vi "Dashboard Main.vi"() -> ()   [LabVIEW 2018]
uses:
  <vilib>/Utility/miscctls.llb/LVRowAndColumnTypeDef.ctl
  <vilib>/event_ctls.llb/eventvkey.ctl
  <vilib>/Rock Robotics/WPI/Dashboard/WPI_DashboardLogging Global.vi
  <vilib>/Rock Robotics/Network Tables/NT Read Numeric Array.vi
  <vilib>/Utility/inputDevices.llb/keyboardAcquire.vi
panel:
  in  "Camera Settings Right":T1={"Frame Rate"=30, "Compression"=30, "Size"=1, "DB Camera Config"=FALSE} {"Frame Rate" scale=1.0..30.0; "Compression" scale=100.0..-1.0; "Size" items=["640x480", "320x240", "160x120"]}
  in  "Camera Name Right":string(combo)="No Camera Selection"
  out "Camera Perf":string
  in  "Camera Settings":T1={"Frame Rate"=30, "Compression"=30, "Size"=1, "DB Camera Config"=FALSE} {"Frame Rate" scale=1.0..30.0; "Compression" scale=100.0..-1.0; "Size" items=["640x480", "320x240", "160x120"]}
  in  "TCP":refnum<k5>
  in  "Rec Mode":enum32{"Stop", "Record", "Playback"}(radio)
  out "Robot IP":string
  out "Image Message":string="Timeout in Camera Communications"
  in  "Dashboard Tab":T2(tab)
  in  "Select Auto":string(combo)="Select Autonomous ..."
  out "NT Connection":bool
  out "MotorChart R":cluster{"Numeric":dbl, "Numeric":dbl}(graph)
  out "MotorChart L":cluster{"Numeric":dbl, "Numeric":dbl}(graph)
  out "MotorSliders R":cluster{"MotorSlide1":dbl, "MotorSlide2":dbl} {"MotorSlide2" scale=-1.0..1.0 scale format="%#_2e"; "MotorSlide1" scale=-1.0..1.0 scale format="%#_2e"}
  out "MotorSliders L":cluster{"MotorSlide1":dbl, "MotorSlide2":dbl} {"MotorSlide2" scale=-1.0..1.0 scale format="%#_2e"; "MotorSlide1" scale=-1.0..1.0 scale format="%#_2e"}
  out "Gyro":dbl(knob) scale=0.0..360.0
  out "JS1 Z":dbl(slide) scale=-1.0..1.0 scale format="%#_2e"
  out "JS1 Graph":cluster{"X":dbl, "Y":dbl}[](graph)
  out "JS1 Buttons":T3
  out "JS2 Z":dbl(slide) scale=-1.0..1.0 scale format="%#_2e"
  out "JS2 Graph":cluster{"X":dbl, "Y":dbl}[](graph)
  out "JS2 Buttons":T3
  out "Mode":T4(ring)=enum."Auto Disabled"
  out "Right Camera Perf":cluster{"Bandwidth (Mbps)":dbl, "FPS":dbl}
  out "Camera Image Right":T5(plugin-control)
  in  "DB/String 9":string
  in  "DB/String 8":string
  in  "DB/String 7":string
  in  "DB/String 6":string
  in  "DB/String 5":string
  in  "DB/String 4":string
  in  "DB/String 3":string
  in  "DB/String 2":string
  in  "DB/String 1":string
  in  "DB/String 0":string
  in  "DB/Slider 0":dbl(slide) scale=0.0..5.0
  in  "DB/Slider 1":dbl(slide) scale=0.0..5.0
  in  "DB/Slider 2":dbl(slide) scale=0.0..5.0
  in  "DB/Slider 3":dbl(slide) scale=0.0..5.0
  out "DB/LED 3":bool
  out "DB/LED 2":bool
  out "DB/LED 1":bool
  out "DB/LED 0":bool
  in  "DB/Button 3":bool
  in  "DB/Button 2":bool
  in  "DB/Button 1":bool
  in  "DB/Button 0":bool caption="New Name"
  in  "Remove Point":bool
  in  "Add Point":bool
  out "XY Graph":cluster{"X":dbl, "Y":dbl}[](graph)
  in  "Interpolation Method":i32(ring)=1 items=["nearest", "linear", "spline", "cubic Hermite", "Lagrange"]
  in  "Test Slider":dbl(slide) scale=0.0..100.0 scale format="%#_3g"
  in  "On/Off":bool caption="Solenoid"
  in  "Test Name":u16(ring) items=["Select the test to run..."]
  in  "Test Tree":string(tree)
  in  "Motor":cluster{"Value":dbl, "Enable":bool} {"Value" scale=-1.0..1.0 scale format="%#_3g"}
  out "Progress":T6 {"Test Progress" scale=0.0..100.0}
  in  "Rev/Fwd":cluster{"Forward":bool, "Reverse":bool}
  in  "Test Ring":u16(ring) items=["Monochrome", "Color"]
  out "Cmd Status":string
  in  "Execute Command":bool
  in  "Command Params":string[][](table)
  in  "Command Selection":i32(listbox)
  in  "CheckList":i32(listbox)
  out "Tree":string(tree)
  out "Camera Image":T5(plugin-control)
  out "Background":bool
  in  "Camera Name":string(combo)="No Camera Selection"
  # "HW"
  # "HW"
  # "Joysticks"
  # "Raw Input"
  # "Proccessed"
  # "Drive Motors"
  # "Front"
  # "Right"
  # "Left"
  # "Back"
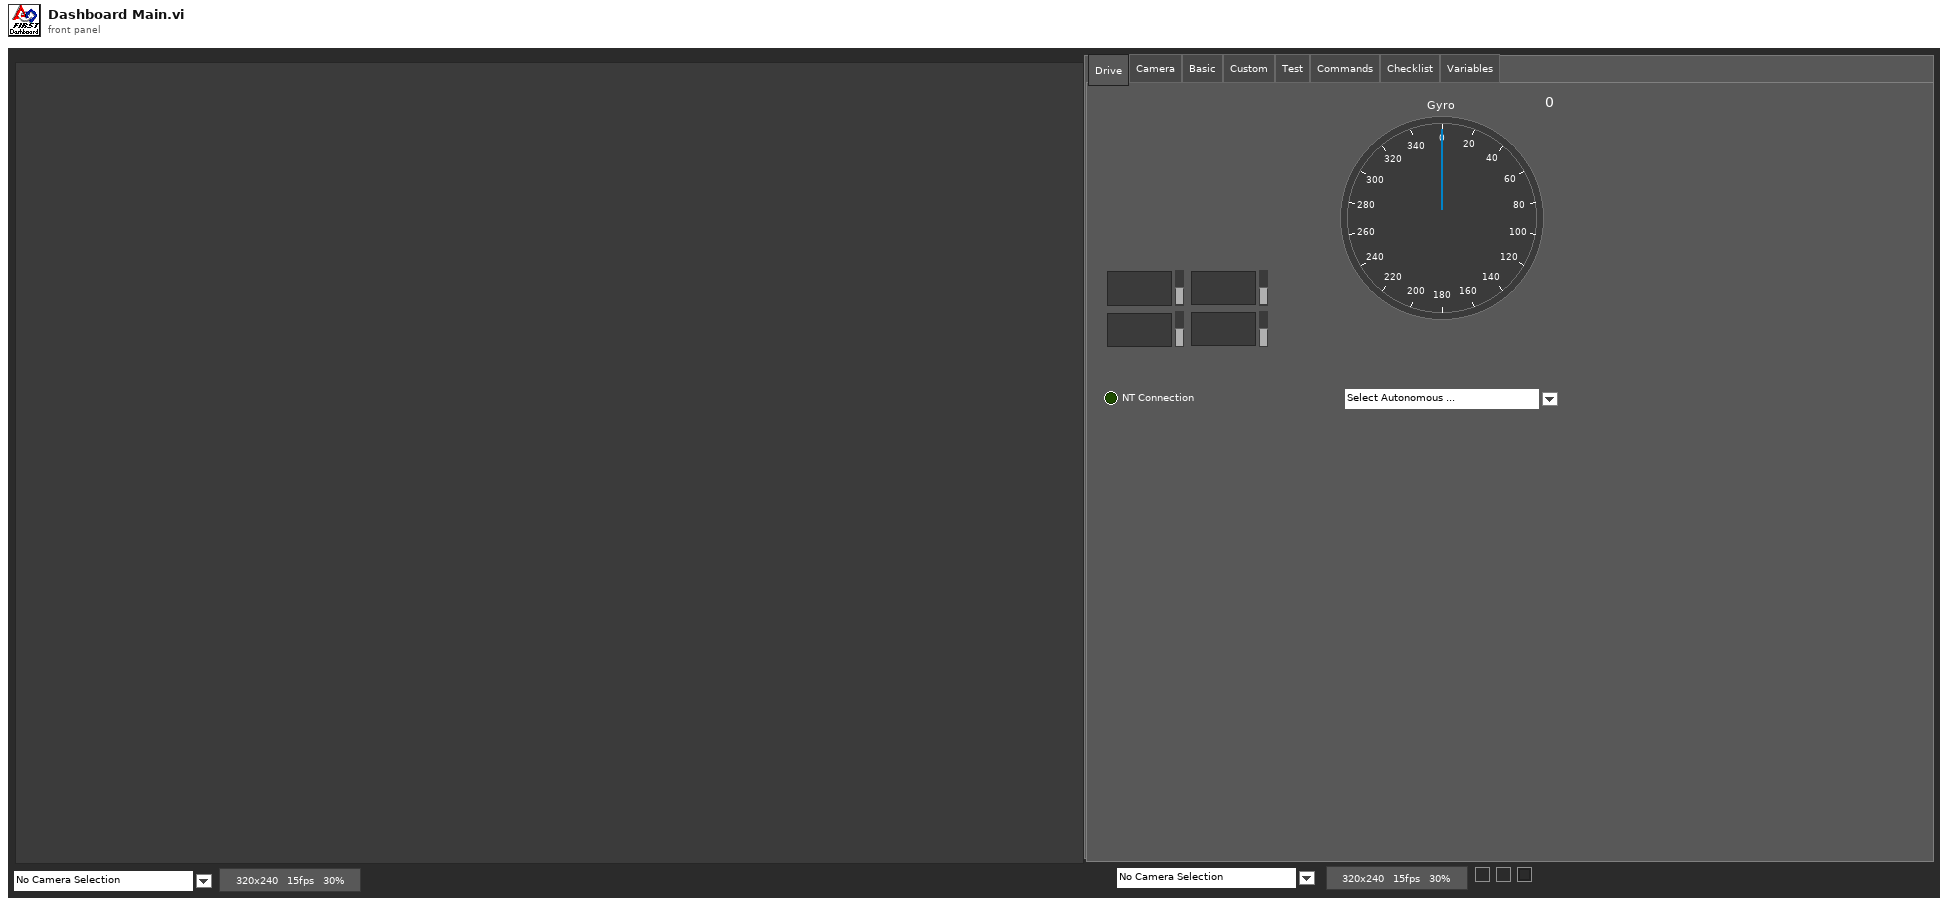
[diagram p1: front panel]
types:
  T1 = cluster{"Frame Rate":i32, "Compression":i32, "Size":u16, "DB Camera Config":bool}
  T2 = enum32{"Drive", "Camera", "Basic", "Custom", "Test", "Commands", "Checklist", "Variables"}
  T3 = cluster{bool, bool, bool, bool, bool, bool, bool, bool, bool, bool, bool, bool}
  T4 = enum8{"Tele-Op Disabled", "Tele-Op Enabled", "Auto Disabled", "Auto Enabled", "Test Disabled", "Test Enabled", "Disconnected", "No Code", "E-Stop"}
  T5 = typedef "IMAQ Image.ctl" = refnum<image>
  T6 = cluster{"Test Progress":u8, "Test Progress Text":string}
  T7 = cluster{"Save Path":path, "Interval (s)":dbl, "Keep":i32}
  T8 = typedef "Image Type" = u32
  T9 = cluster{"IDs":cluster{"RPC field ID":u16, "Unique ID":u16}, "String":string}
  T10 = cluster{"Camera Image":refnum<vi>, "Dashboard Tab":refnum<vi>, "Background":refnum<vi>, "Rec Mode":refnum<vi>, "Test Slider":refnum<vi>, "On/Off ":refnum<vi>, "Test Ring":refnum<vi>, "Rev/Fwd":refnum<vi>, "Test Name":refnum<vi>, "Motor":refnum<vi>, "Progress":refnum<vi>, "CheckList":refnum<vi>, "Tree":refnum<vi>, "Test Tree":refnum<vi>, "Command Params":refnum<vi>, "Command Selection":refnum<vi>, "Execute Command":refnum<vi>, "Cmd Status":refnum<vi>, "Camera Settings":refnum<vi>, "Camera Name":refnum<vi>, "Camera Perf":refnum<vi>, "Camera Settings Right":refnum<vi>, "Camera Name Right":refnum<vi>, "Camera Image Right":refnum<vi>}
  T11 = cluster{"Global Rectangle":i32[], "Contours":cluster{"Contour Type":u32, "ROI Type":u32, "Points":i32[]}[]}
  T12 = cluster{"Camera Name":string, string, "Saved DB Images Info":cluster{"Save Path":path, "Interval (s)":dbl, "Keep":i32}}
  T13 = cluster{"Camera Name Right":string, string, "Saved DB Images Info":cluster{"Save Path":path, "Interval (s)":dbl, "Keep":i32}}
  T14 = cluster{"Operation":enum16{"Update", "Clear"}, "Color Box":u32}[]
  T15 = typedef "eventvkey.ctl" = enum16{"ASCII", "Enter", "Return", "Shift", "Ctrl", "Alt", "Cmd", "Opt", "Caps", "NumLock", "Clear", "Break", "Up", "Down", "Left", "Right", "Insert", "Delete", "Home", "End", "PageUp", "PageDown", "Escape", "Help", "Pause", "ScrollLock", "F1", "F2", "F3", "F4", "F5", "F6", "F7", "F8", "F9", "F10", "F11", "F12", "F13", "F14", "F15", "F16", "F17", "F18", "F19", "F20", "F21", "F22", "F23", "F24", "Play", "VolumeUp", "VolumeDown", "Mute", "Two Byte Char"}
  T16 = cluster{"Image Size":bool, "Image Type":bool, "Pixel Value":bool, "ROI Information":bool, "Zoom Factor":bool}
  T17 = cluster{"Operation":enum16{"Update", "Clear"}, "Color Box":u32}
  T18 = typedef "LVRowAndColumnTypeDef.ctl" = cluster{"Row":i32, "Column":i32}
  T19 = cluster{"Shift":bool, "Ctrl":bool, "Alt":bool, "Cmd":bool, "Opt":bool}
  T20 = cluster{"Error Strings":string, "Disable Counts":cluster{u16, u16}, "Rail Faults":cluster{u16, u16, u16}, "Robot IP":string, "DB Mode":u8, "Event Info":cluster{"Name":string, "Type":u8, "Number":u16, "Replay":u8}}
  T21 = cluster{"Storage":cluster{"Disk Free":u64, "RAM Block":u32, "RAM free":u32}, "CPU Utilization":cluster{"CPU % ISR":sgl, "CPU % Time Crit":sgl, "CPU % Timed Str":sgl, "CPU % High":sgl, "CPU % Above":sgl, "CPU % Normal":sgl, "CPU % Low":sgl}, "CAN":cluster{"% Bus Utilization":sgl, "Bus Off Cnt":u32, "TX_FIFO Full Cnt":u32, "Receive Error Cnt":u8, "Transmit Error Cnt":u8}, "HID":cluster{"HID Outputs":u32, "Rumble Low":u16, "Rumble High":u16}[]}
  T22 = cluster{"Status bits":cluster{"Test Mode":bool, "Autonomous":bool, "Enabled":bool, "Code Start":bool, "Brownout":bool, "Reserved 2":bool, "Reserved 3":bool, "E-Stop":bool}, "Code Trace":cluster{"Disabled":bool, "TeleOp":bool, "Auto":bool, "Test":bool}, "Controller Type":enum16{"unknown", "cRIO", "roboRio"}, "Code?":enum16{"unknown", "noCode", "code"}, "Battery V":dbl}
  T23 = cluster{"Control Bits":cluster{"TestMode":bool, "Autonomous":bool, "Enabled":bool, "FMS Present":bool, bool, bool, bool, "E-Stop":bool}, "Team Station ":u8, "Countdown":sgl, "Joystick Values":cluster{"Axes":dbl[], "Buttons":bool[], "POVs":i16[]}[]}
  T24 = cluster{"Axes":dbl[], "Buttons":bool[], "POVs":i16[]}[]
  T25 = cluster{"Axes":dbl[], "Buttons":bool[], "POVs":i16[]}
  T26 = cluster{"Buttons[0]":bool, "Buttons[1]":bool, "Buttons[2]":bool, "Buttons[3]":bool, "Buttons[4]":bool, "Buttons[5]":bool, "Buttons[6]":bool, "Buttons[7]":bool, "Buttons[8]":bool, "Buttons[9]":bool, "Buttons[10]":bool, "Buttons[11]":bool}
  T27 = enum16{"0", "1", "2", "3", "4", "5", "6", "7", "8", "9", "A", "B", "C", "D", "E", "F", "G", "H", "I", "J", "K", "L", "M", "N", "O", "P", "Q", "R", "S", "T", "U", "V", "W", "X", "Y", "Z", "F1", "F2", "F3", "F4", "F5", "F6", "F7", "F8", "F9", "F10", "F11", "F12", "F13", "F14", "F15", "ADD", "BACK", "BACKSLASH", "CAPITAL", "COMMA", "DECIMAL", "DELETE", "DIVIDE", "DOWN", "END", "EQUALS", "ESCAPE", "GRAVE (`)", "HOME", "INSERT", "LBRACKET", "LCONTROL", "LEFT", "L ALT", "LSHIFT", "LWIN", "MINUS", "MULTIPLY", "NEXT", "NUMLOCK", "NUMPAD_0", "NUMPAD_1", "NUMPAD_2", "NUMPAD_3", "NUMPAD_4", "NUMPAD_5", "NUMPAD_6", "NUMPAD_7", "NUMPAD_8", "NUMPAD_9", "PAUSE", "PERIOD", "PRIOR (PG UP)", "RBRACKET", "RCONTROL", "RETURN", "RIGHT", "R ALT", "RSHIFT", "RWIN", "SCROLL", "SEMICOLON", "SLASH", "SPACE", "SUBTRACT", "TAB", "UP", "ENTER (num pad)", "' (quote)"}[]
  T28 = enum16{"0", "1", "2", "3", "4", "5", "6", "7", "8", "9", "A", "B", "C", "D", "E", "F", "G", "H", "I", "J", "K", "L", "M", "N", "O", "P", "Q", "R", "S", "T", "U", "V", "W", "X", "Y", "Z", "F1", "F2", "F3", "F4", "F5", "F6", "F7", "F8", "F9", "F10", "F11", "F12", "F13", "F14", "F15", "ADD", "BACK", "BACKSLASH", "CAPITAL", "COMMA", "DECIMAL", "DELETE", "DIVIDE", "DOWN", "END", "EQUALS", "ESCAPE", "GRAVE (`)", "HOME", "INSERT", "LBRACKET", "LCONTROL", "LEFT", "L ALT", "LSHIFT", "LWIN", "MINUS", "MULTIPLY", "NEXT", "NUMLOCK", "NUMPAD_0", "NUMPAD_1", "NUMPAD_2", "NUMPAD_3", "NUMPAD_4", "NUMPAD_5", "NUMPAD_6", "NUMPAD_7", "NUMPAD_8", "NUMPAD_9", "PAUSE", "PERIOD", "PRIOR (PG UP)", "RBRACKET", "RCONTROL", "RETURN", "RIGHT", "R ALT", "RSHIFT", "RWIN", "SCROLL", "SEMICOLON", "SLASH", "SPACE", "SUBTRACT", "TAB", "UP", "ENTER (num pad)", "' (quote)"}
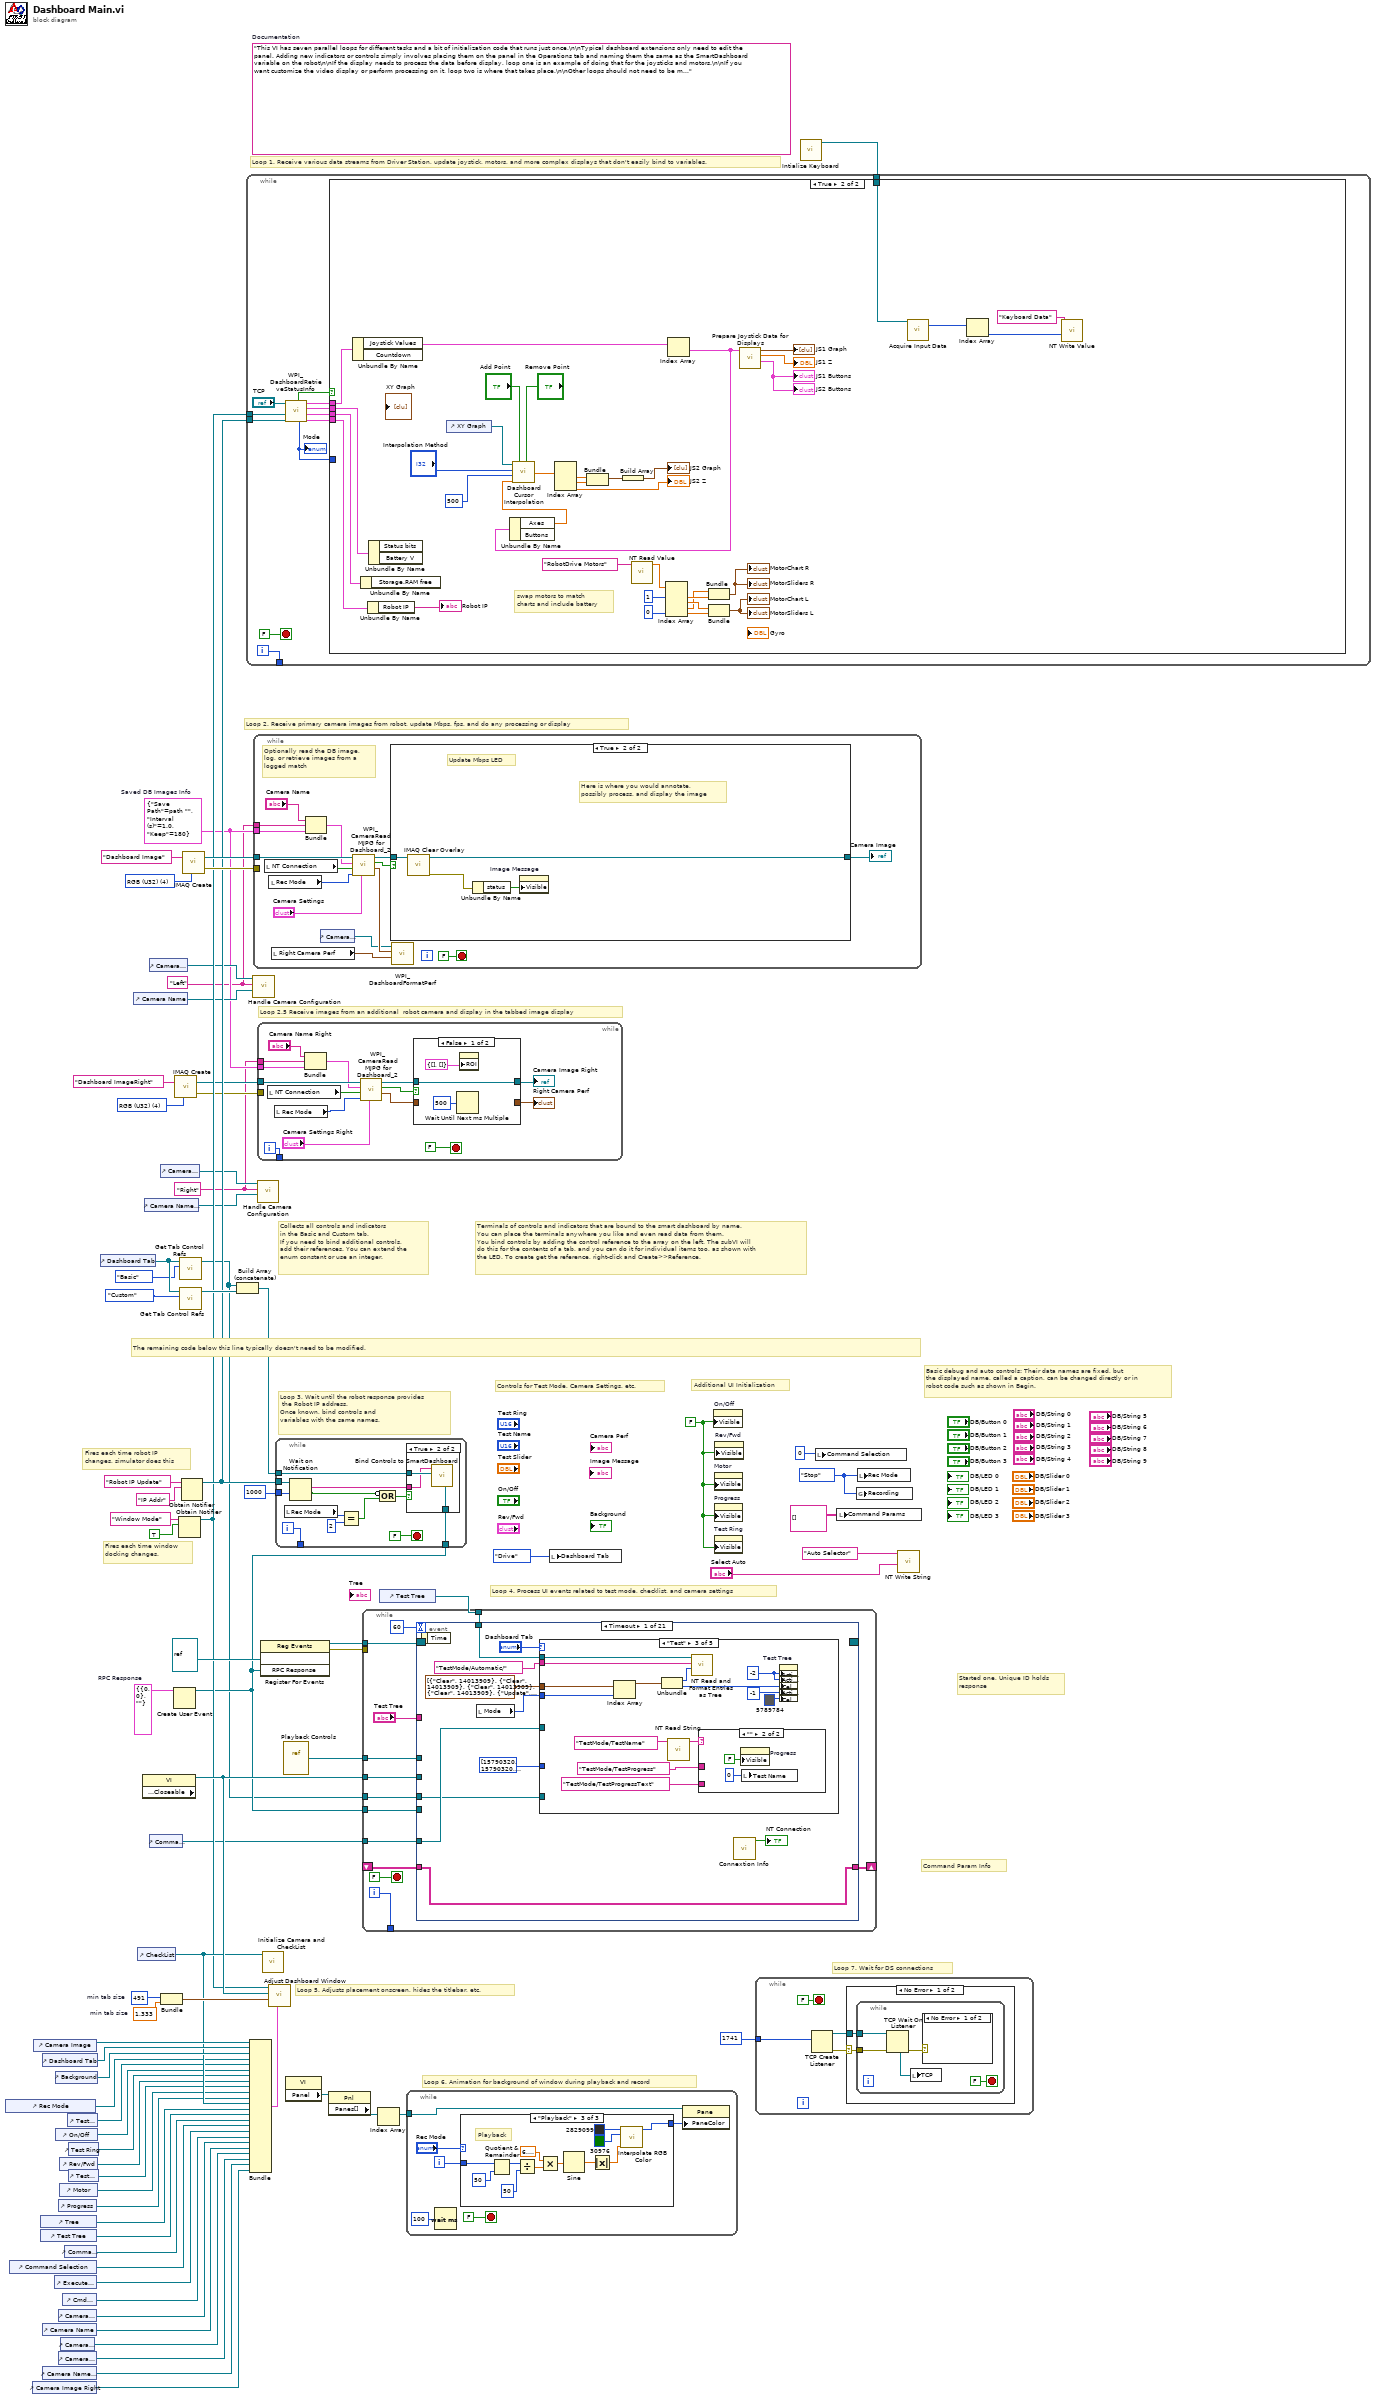
[diagram p0: block diagram]
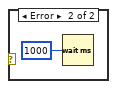
[diagram p3: hidden frame]
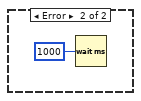
[diagram p4: hidden frame]
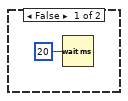
[diagram p5: hidden frame]
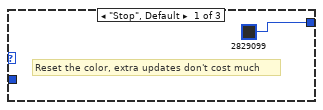
[diagram p6: hidden frame]
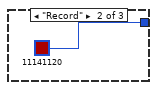
[diagram p7: hidden frame]
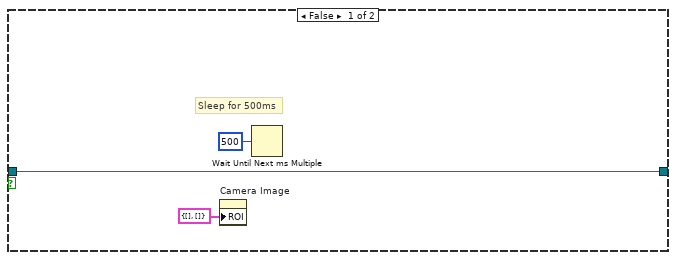
[diagram p9: hidden frame]
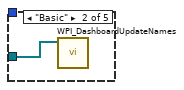
[diagram p11: hidden frame]
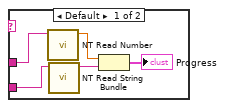
[diagram p12: hidden frame]
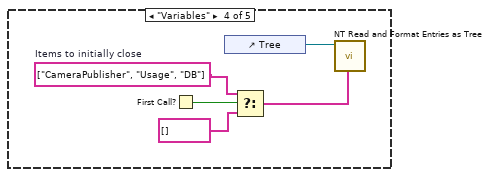
[diagram p13: hidden frame]
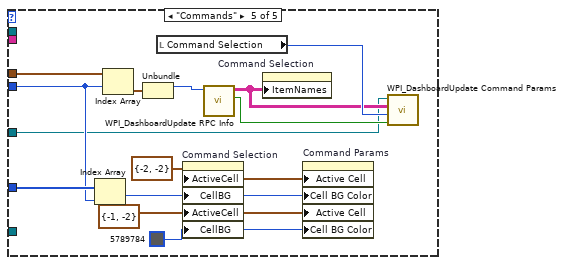
[diagram p14: hidden frame]
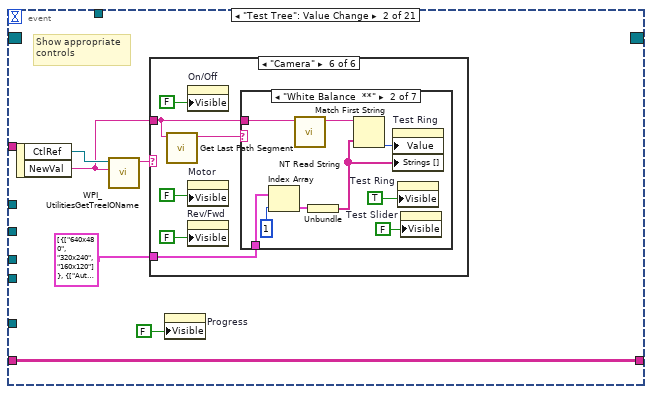
[diagram p15: hidden frame]
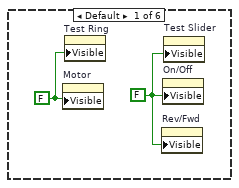
[diagram p16: hidden frame]
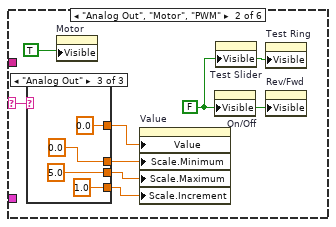
[diagram p17: hidden frame]
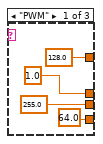
[diagram p18: hidden frame]
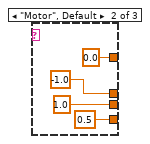
[diagram p19: hidden frame]
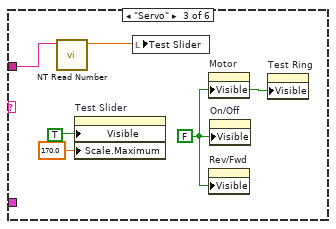
[diagram p20: hidden frame]
diagram:
  w4 = T7 {"Save Path"=path "", "Interval (s)"=1.0, "Keep"=180}  # Saved DB Images Info
  w3 = "Right"
  w2 = "Left"
  w14 = T8 4 items=["Grayscale (U8)", "Grayscale (I16)", "Grayscale (SGL)", "Complex (CSG)", "RGB (U32)", "HSL (U32)", "RGB (U64)"] ("Image Type")
  w30 = T9 {"IDs"={"RPC field ID"=0, "Unique ID"=0}, "String"=""}  # RPC Response
  w53 = 491  # min tab size
  w52 = 1.333  # min tab size
  w60 = enum32{"Stop", "Record", "Playback"}."Stop" ("Rec Mode")
  w37 = FALSE ("Visible")
  (unwired) "This VI has seven parallel loops for different tasks and a bit of initialization code that runs just once.\n\nTypical dashboard extensions only need to edit the panel. Adding new indicators or controls simply involves placing them on the panel in the Operations tab and naming them the same as the SmartDashboard variable on the robot\n\nIf the display needs to process the data before display, loop one is an example of doing that for the joysticks and motors.\n\nIf you want customize the video display or perform processing on it, loop two is where that takes place.\n\nOther loops should not need to be modified. They are pretty standard, and document the task they perform."  # Documentation
  w77 = T8 4 items=["Grayscale (U8)", "Grayscale (I16)", "Grayscale (SGL)", "Complex (CSG)", "RGB (U32)", "HSL (U32)", "RGB (U64)"] ("Image Type")
  # "Loop 2.5 Receive images from an additional  robot camera and display in the tabbed image display"
  # "Command Param Info"
  # "Started one, Unique ID holds\nresponse"
  # "Loop 7. Wait for DS connections"
  # "Basic debug and auto controls: Their data names are fixed, but\nthe displayed name, called a caption, can be changed directly or in\nrobot code such as shown in Begin."
  # "Controls for Test Mode, Camera Settings, etc."
  # "Additional UI Initialization"
  # "Loop 6. Animation for background of window during playback and record"
  # "Fires each time robot IP\nchanges, simulator does this"
  # "Fires each time window\ndocking changes."
  # "Collects all controls and indicators\nin the Basic and Custom tab.\nIf you need to bind additional controls,\nadd their references. You can extend the\nenum constant or use an integer."
  # "The remaining code below this line typically doesn't need to be modified."
  # "Loop 4. Process UI events related to test mode, checklist, and camera settings"
  # "Terminals of controls and indicators that are bound to the smart dashboard by name.\nYou can place the terminals anywhere you like and even read data from them.\nYou bind controls by adding the control reference to the array on the left. The subVI will\ndo this for the contents of a tab, and you can do it for individual items too, as shown with\nthe LED. To create get the reference, right-click and Create>>Reference."
  # "Loop 3. Wait until the robot response provides\n the Robot IP address.\nOnce known, bind controls and\nvariables with the same names."
  # "Loop 5. Adjusts placement onscreen, hides the titlebar, etc."
  # "Loop 1. Receive various data streams from Driver Station, update joystick, motors, and more complex displays that don't easily bind to variables."
  # "Loop 2. Receive primary camera images from robot, update Mbps, fps, and do any processing or display"
  n1 = control-ref of="Rec Mode"() -> (w43:refnum<vi>)
  n2 = control-ref of="Command Selection"() -> (w29:refnum<vi>)
  n3 = control-ref of="Camera Image Right"() -> (w7:refnum<vi>)
  n4 = control-ref of="Camera Image"() -> (w55:refnum<vi>)
  n5 = control-ref of="Tree"() -> (w47:refnum<vi>)
  n6 = control-ref of="Test Tree"() -> (w46:refnum<vi>)
  n7 = control-ref of="Dashboard Tab"() -> (w54:refnum<vi>)
  n8 = control-ref of="Camera Name"() -> (w20:refnum<vi>)
  n9 = control-ref of="Camera Name Right"() -> (w8:refnum<vi>)
  n10 = control-ref of="Execute Command"() -> (w31:refnum<vi>)
  n11 = control-ref of="Background"() -> (w50:refnum<vi>)
  n12 = control-ref of="On/Off"() -> (w41:refnum<vi>)
  n13 = control-ref of="Progress"() -> (w38:refnum<vi>)
  n14 = control-ref of="Camera Settings"() -> (w21:refnum<vi>)
  n15 = control-ref of="Camera Settings Right"() -> (w9:refnum<vi>)
  n16 = control-ref of="Rev/Fwd"() -> (w39:refnum<vi>)
  n17 = control-ref of="Motor"() -> (w44:refnum<vi>)
  n18 = control-ref of="Camera Perf"() -> (w19:refnum<vi>)
  n19 = control-ref of="Cmd Status"() -> (w25:refnum<vi>)
  n20 = control-ref of="Command Params"() -> (w32:refnum<vi>)
  n21 = control-ref of="Test Slider"() -> (w42:refnum<vi>)
  n22 = control-ref of="Test Ring"() -> (w40:refnum<vi>)
  n23 = control-ref of="Test Name"() -> (w45:refnum<vi>)
  n24 = control-ref of="Dashboard Tab"() -> (w58:refnum<vi>)
  n25 = control-ref of="Camera Name"() -> (w22:refnum<vi>)
  n26 = control-ref of="CheckList"() -> (w48:refnum<vi>)
  n27 = property class="VI" props=["Front Panel.Closeable"]() -> (reference out=w59:refnum<vi>)  [unwired: 2 in, 2 out]
  n28 = control-ref of="Camera Name Right"() -> (w10:refnum<vi>)
  n29 = control-ref of="Camera Settings"() -> (w23:refnum<vi>)
  n30 = control-ref of="Command Params"() -> (w24:refnum<vi>)
  n31 = control-ref of="Camera Settings Right"() -> (w11:refnum<vi>)
  n32 = Bundle("min tab size"=w53, "min tab size"=w52) -> (w51:cluster{"min tab size":i32, "min tab size":dbl})  [unwired: 1 in]
  n33 = Create User Event(user event datatype=w30) -> (user event=w26:refnum<user-event>)  [unwired: 1 in, 1 out]
  n34 = call "IMAQ Create"("Image Name"="Dashboard ImageRight", "Image Type"=w14) -> ("New Image"=w13:T5, "error out"=w12:errorcluster)  [unwired: 2 in, 1 out]
  n35 = Obtain Notifier(name (unnamed)="Window Mode", notification data type=TRUE) -> (notifier out=w35:refnum<notifier>)  [unwired: 2 in, 2 out]
  n36 = call <vilib>:"Get Tab Control Refs.vi"("Page Index"=T2."Basic" ("Dashboard Tab"), "TabControl in"=w58) -> ("ControlsOnPage"=w18:refnum<vi>[])  [unwired: 9 in]
  n37 = call <vilib>:"Get Tab Control Refs.vi"("Page Index"=T2."Custom" ("Dashboard Tab"), "TabControl in"=w58) -> ("ControlsOnPage"=w57:refnum<vi>[])  [unwired: 9 in]
  n38 = Obtain Notifier(name (unnamed)="Robot IP Update", notification data type="IP Addr" ("name (unnamed)")) -> (notifier out=w36:refnum<notifier>)  [unwired: 2 in, 2 out]
  n39 = call "IMAQ Create"("Image Name"="Dashboard Image", "Image Type"=w77) -> ("New Image"=w75:T5, "error out"=w74:errorcluster)  [unwired: 2 in, 1 out]
  n40 = Build Array (concatenate)(w18, w57) -> (w56:refnum<vi>[])
  n41 = Bundle("Camera Image"=w55, "Dashboard Tab"=w54, "Background"=w50, "Rec Mode"=w43, "Test Slider"=w42, "On/Off"=w41, "Test Ring"=w40, "Rev/Fwd"=w39, "Test Name"=w45, "Motor"=w44, "Progress"=w38, "CheckList"=w48, "Tree"=w47, "Test Tree"=w46, "Command Params"=w32, "Command Selection"=w29, "Execute Command"=w31, "Cmd Status"=w25, "Camera Settings"=w21, "Camera Name"=w20, "Camera Perf"=w19, "Camera Settings Right"=w9, "Camera Name Right"=w8, "Camera Image Right"=w7) -> (w49:T10)  [unwired: 1 in]
  n42 = call "Handle Camera Configuration.vi"("CameraNameRef"=w22, "Display Name"=w2, "ClusterRef"=w23) -> ()  [unwired: 9 in]
  n43 = while {
    tunnel: w75 -> [w91]
    tunnel: w74 -> [_]
    tunnel: w4 -> [w84]
    tunnel: w2 -> [w81]
    stop <- FALSE stop-if-true
    # "Optionally read the DB image,\nlog, or retrieve images from a\nlogged match"
    n44 = local read "NT Connection"() -> (w85:bool)
    n45 = local read "Rec Mode"() -> (w88:enum32{"Stop", "Record", "Playback"})
    n46 = local read "Right Camera Perf"() -> (w79:cluster{"Bandwidth (Mbps)":dbl, "FPS":dbl})
    n47 = Bundle("Camera Name"="Camera Name", w81, "Saved DB Images Info"=w84) -> (w83:T12)  [unwired: 1 in]
    n48 = control-ref of="Camera Perf"() -> (w78:refnum<vi>)
    n49 = call <vilib>:"WPI_CameraRead MJPG for Dashboard_2.vi"("Camera Settings"="Camera Settings", "Rec Mode"=w88, "NT Connection"=w85, "Capture Info"=w83, "Image in"=w91) -> ("perf info"=w80:cluster{"Bandwidth (Mbps)":dbl, "fps":dbl}, "Active"=w89:bool, "Image\\ out"=w90:T5)  [unwired: 4 in]
    n50 = case shown="True" w89 {
      tunnel: w90 -> [w94 w97]
      tunnel: [w94 w96] -> w86
      frame False {
        # "Sleep for 500ms"
        n51 = property on="Camera Image" class="ImageControl"("ROI"=T11 {"Global Rectangle"=[], "Contours"=[]}) -> ()  [unwired: 2 in, 2 out]
        n52 = Wait Until Next ms Multiple(millisecond multiple=u32 500) -> ()  [unwired: 1 out]
      }
      frame True {
        # "Here is where you would annotate,\npossibly process, and display the image"
        # "Update Mbps LED"
        n53 = call "IMAQ Clear Overlay"("Image"=w97) -> ("error out"=w98:errorcluster, "Image Out"=w96:T5)  [unwired: 2 in, 7 out]
        n54 = Unbundle By Name(w98) -> ("status"=w99:bool)
        n55 = property on="Image Message" class="Str"("Visible"=w99) -> ()  [unwired: 2 in, 2 out]
      }
    }
    "Camera Image" <- w86
    n56 = call <vilib>:"WPI_DashboardFormatPerf.vi"("Right Camera Perf"=w79, "Performance"=w80, "String in"=w78) -> ()  [unwired: 9 in]
  }
  n57 = call "Handle Camera Configuration.vi"("CameraNameRef"=w10, "Display Name"=w3, "ClusterRef"=w11) -> ()  [unwired: 9 in]
  n58 = while {
    tunnel: w13 -> [w114]
    tunnel: w12 -> [_]
    tunnel: [w109] -> _
    tunnel: w4 -> [w105]
    tunnel: w3 -> [w102]
    i -> [w109]
    stop <- FALSE stop-if-true
    n59 = local read "NT Connection"() -> (w106:bool)
    n60 = local read "Rec Mode"() -> (w113:enum32{"Stop", "Record", "Playback"})
    n61 = Bundle("Camera Name Right"="Camera Name Right", w102, "Saved DB Images Info"=w105) -> (w104:T13)  [unwired: 1 in]
    n62 = call <vilib>:"WPI_CameraRead MJPG for Dashboard_2.vi"("Camera Settings"="Camera Settings Right", "Rec Mode"=w113, "NT Connection"=w106, "Capture Info"=w104, "Image in"=w114) -> ("perf info"=w100:cluster{"Bandwidth (Mbps)":dbl, "fps":dbl}, "Active"=w108:bool, "Image\\ out"=w111:T5)  [unwired: 4 in]
    n63 = case shown="False" w108 {
      tunnel: w111 -> [w116 w119]
      tunnel: [w116 w119] -> w107
      tunnel: [_ w118] -> w101
      tunnel: w100 -> [_ w118]
      frame False {
        n64 = Wait Until Next ms Multiple(millisecond multiple=u32 500) -> ()  [unwired: 1 out]
        n65 = property on="Camera Image Right" class="ImageControl"("ROI"=T11 {"Global Rectangle"=[], "Contours"=[]}) -> ()  [unwired: 2 in, 2 out]
      }
      frame True {
      }
    }
    "Camera Image Right" <- w107
    "Right Camera Perf" <- w101
  }
  n66 = register-events(refnum<vi> refnum, w26) -> (reference out=w64:refnum<event-registration>, error out=w63:errorcluster)  [unwired: 2 in]
  n67 = call "Initialize Camera and CheckList.vi"("ListBox in"=w48) -> ()  [unwired: 11 in]
  n68 = call "Adjust Dashboard Window.vi"("Sizing Refnums"=w49, "Size Constraints"=w51, "VI"=w59, "WIn Mode"=w35) -> ()  [unwired: 8 in]
  n69 = while {
    tunnel: w56 -> [w131]
    tunnel: w36 -> [w129]
    tunnel: [w127] -> _
    tunnel: u32 1000 ("milliseconds to wait") -> [w126]
    tunnel: w26 -> [w120]
    i -> [w127]
    stop <- FALSE stop-if-true
    n70 = local read "Rec Mode"() -> (w122:enum32{"Stop", "Record", "Playback"})
    n71 = Wait on Notification(notifier=w129, timeout in ms (-1)=w126) -> (notification=w128:string, timed out?=w124:bool)  [unwired: 2 in, 2 out]
    n72 = Equal?(x=w122, y=u16 2 ("Rec Mode")) -> (x = y?=w123:bool)
    n73 = Compound Arithmetic op=OR(invert w124, w123) -> (w125:bool)
    n74 = case shown="True" w125 {
      tunnel: w131 -> [_ w134]
      tunnel: w128 -> [_ w133]
      tunnel: w120 -> [_ w132]
      frame False {
      }
      frame True {
        n75 = call <vilib>:"Bind Controls to SmartDashboard.vi"("RPC ref"=w132, "Bound Control Refs"=w134, "Server IP Address"=w133) -> ()  [unwired: 9 in]
      }
    }
  }
  n76 = vi-ref "Playback Controls.vi"() -> (w65:refnum<vi>)
  n77 = property class="VI"() -> ("Panel"=w67:refnum<vi>)  [unwired: 2 in, 2 out]
  n78 = property class="Pnl"(reference=w67) -> ("Panes[]"=w68:refnum<vi>[])  [unwired: 1 in, 2 out]
  n79 = Index Array(array=w68) -> (element=w66:refnum<vi>)  [unwired: 1 in]
  n80 = control-ref of="Test Tree"() -> (w69:refnum<vi>)
  n81 = while {
    tunnel: [w144] -> _
    tunnel: w69 -> [w143]
    tunnel: w65 -> [w142]
    tunnel: w64 -> [w141]
    tunnel: w63 -> [_]
    tunnel: w59 -> [w140]
    tunnel: w26 -> [w139]
    tunnel: w24 -> [w138]
    shift-right: [w137] -> _
    shift-left: _ -> [w136]
    tunnel: w18 -> [w135]
    i -> [w144]
    stop <- FALSE stop-if-true
    n82 = event shown="[0] Timeout" {
      selector: w141 -> [_ _ _ _ _ _ _ _ _ _ _ _ _ _ _ _ _ _ _ _ _]
      dyn-events: [_ _ _ _ _ _ _ _ _ _ _ _ _ _ _ _ w404 _ _ _ _] -> _
      timeout: u32 60 ("milliseconds to wait") -> [_ _ _ _ _ _ _ _ _ _ _ _ _ _ _ _ _ _ _ _ _]
      tunnel: w143 -> [w156 _ _ _ _ _ _ _ _ _ _ _ _ _ _ _ _ _ _ _ _]
      tunnel: "Test Tree" -> [_ _ _ _ _ _ _ _ _ _ _ w371 w379 w381 w385 w393 _ _ _ _ _]
      tunnel: w142 -> [_ _ _ _ _ _ _ _ _ _ _ _ _ _ _ _ w406 _ w424 _ _]
      tunnel: w140 -> [_ _ _ _ _ _ _ _ _ _ _ _ _ _ _ _ w402 _ _ _ _]
      tunnel: w139 -> [_ _ _ _ _ _ _ _ _ _ _ _ _ _ _ _ w400 _ _ _ _]
      tunnel: w138 -> [w151 _ _ _ _ _ w322 _ _ _ _ _ _ _ _ _ _ _ _ _ _]
      tunnel: [w150 w199 w301 w306 w315 w319 w320 w329 w339 w346 w358 w370 w377 w380 w384 w392 w399 w419 w421 w425 w438] -> w137
      tunnel: w136 -> [w150 w199 w301 w306 w315 w319 w320 _ _ w346 w358 w370 w377 w380 w384 w392 w399 w419 w421 w425 w438]
      tunnel: w135 -> [w148 _ _ _ _ _ _ _ _ _ _ _ _ _ _ _ _ _ _ _ _]
      event Timeout {
        n83 = event-data() -> ()  [unwired: 1 in, 1 out]
        n84 = local read "Mode"() -> (w153:T4)
        n85 = case shown="\"Test\"" "Dashboard Tab" {
          tunnel: w156 -> [_ _ w172 _ _]
          tunnel: "TestMode/Automatic/" ("Name Pattern") -> [_ _ w171 _ _]
          tunnel: T14 [{"Operation"=enum."Clear", "Color Box"=14013909}, {"Operation"=enum."Clear", "Color Box"=14013909}, {"Operation"=enum."Clear", "Color Box"=14013909}, {"Operation"=enum."Clear", "Color Box"=14013909}, {"Operation"=enum."Update", "Color Box"=14013909}, {"Operation"=enum."Update", "Color Box"=16777215}, {"Operation"=enum."Clear", "Color Box"=14013909}, {"Operation"=enum."Clear", "Color Box"=14013909}, {"Operation"=enum."Clear", "Color Box"=14013909}] -> [_ _ w164 _ w192]
          tunnel: w153 -> [_ _ w163 _ w191]
          tunnel: u32[] [15790320, 15790320, 15790320, 15790320, 16777215, 16777215, 15790320, 15790320, 15790320] -> [_ _ _ _ w197]
          tunnel: w151 -> [_ _ _ _ w185]
          tunnel: w148 -> [_ w158 _ _ _]
          frame "Custom", Default {
          }
          frame "Basic" {
            n86 = call <vilib>:"WPI_DashboardUpdateNames.vi"("Controls on Tab"=w158) -> ()  [unwired: 11 in]
          }
          frame "Test" {
            w170 = -2 ("Active Item:Row Number")
            n87 = Index Array(array=w164, index=w163) -> (element=w165:T17)
            n88 = Unbundle(w165) -> ("Operation"=w166:enum16{"Update", "Clear"}, "Color Box"=w167:u32)
            n89 = call <vilib>:"NT Read String.vi"("Name"="TestMode/TestName") -> ("String"=w161:string)  [unwired: 9 in, 1 out]
            n90 = call <vilib>:"NT Read and Format Entries as Tree.vi"("Operation"=w166, "Name Pattern"=w171, "Tree Refnum"=w172) -> ()  [unwired: 7 in, 2 out]
            n91 = case shown="\"\"" w161 {
              tunnel: "TestMode/TestProgress" ("Name") -> [w174 _]
              tunnel: "TestMode/TestProgressText" ("Name") -> [w173 _]
              frame Default {
                n92 = call <vilib>:"NT Read Number.vi"("Name"=w174) -> ("Numeric"=w175:dbl)  [unwired: 9 in, 1 out]
                n93 = call <vilib>:"NT Read String.vi"("Name"=w173) -> ("String"=w176:string)  [unwired: 9 in, 1 out]
                n94 = Bundle("Numeric"=w175, "String"=w176) -> (→"Progress":cluster{"Numeric":dbl, "String":string})  [unwired: 1 in]
              }
              frame "" {
                n95 = property on="Progress" class="Clust (strict)"("Visible"=FALSE) -> ()  [unwired: 2 in, 2 out]
                n96 = local write "Test Name"(u16 0) -> ()
              }
            }
            n97 = property on="Test Tree" class="Tree (strict)"("Active Item Row Number"=w170, "ActiveColNum"=w170, "CellBG"=w167, "Active Item Row Number"=-1 ("Active Item:Row Number"), "CellBG"=u32 5789784 ("Color Box")) -> ()  [unwired: 2 in, 2 out]
          }
          frame "Variables" {
            w182 = string[] ["CameraPublisher", "Usage", "DB"]  # Items to initially close
            n98 = First Call?() -> (First Call?: T/F=w183:bool)
            n99 = control-ref of="Tree"() -> (w184:refnum<vi>)
            n100 = Select(t=w182, s=w183, f=string[] []) -> (s? t:f=w180:string[])
            n101 = call <vilib>:"NT Read and Format Entries as Tree.vi"("Tags to  Close"=w180, "Tree Refnum"=w184) -> ()  [unwired: 8 in, 2 out]
          }
          frame "Commands" {
            w193 = u32 5789784 ("Color Box")
            w194 = T18 {"Row"=-1, "Column"=-2} ("Active Cell:Active Cell")
            w196 = T18 {"Row"=-2, "Column"=-2} ("Active Cell:Active Cell")
            n102 = Index Array(array=w197, index=w191) -> (element=w195:u32)
            n103 = Index Array(array=w192, index=w191) -> (element=w190:T17)
            n104 = Unbundle(w190) -> ("Operation"=w189:enum16{"Update", "Clear"})  [unwired: 1 out]
            n105 = local read "Command Selection"() -> (w188:i32)
            n106 = property on="Command Selection" class="MCListbox (strict)"("ActiveCell"=w196, "CellBG"=w195, "ActiveCell"=w194, "CellBG"=w193) -> ()  [unwired: 2 in, 2 out]
            n107 = call <vilib>:"WPI_DashboardUpdate RPC Info.vi"("Operation"=w189) -> ("update"=w187:bool, "commands"=w186:string[][])  [unwired: 9 in]
            n108 = property on="Command Selection" class="MCListbox (strict)"("ItemNames"=w186) -> ()  [unwired: 2 in, 2 out]
            n109 = property on="Command Params" class="Tbl (strict)"("Active Cell"=w196, "Cell BG Color"=w195, "Active Cell"=w194, "Cell BG Color"=w193) -> ()  [unwired: 2 in, 2 out]
            n110 = call <vilib>:"WPI_DashboardUpdate Command Params.vi"("Update"=w187, "NewVal"=w188, "Commands"=w186, "Param Tbl"=w185) -> ()  [unwired: 7 in, 1 out]
          }
        }
        n111 = call <vilib>:"Connextion Info.vi"() -> ("Connected"=→"NT Connection":bool)  [unwired: 10 in, 1 out]
      }
      event "Test Tree": Value Change {
        # "Show appropriate\ncontrols"
        n112 = event-data() -> ("CtlRef"=w202:refnum<vi>, "NewVal"=w200:string)  [unwired: 1 in]
        n113 = call <vilib>:"WPI_UtilitiesGetTreeIOName.vi"("NewVal"=w200, "TreeControl in"=w202) -> ("I/O Name"=w203:string)  [unwired: 9 in]
        n114 = case shown="\"Camera\"" w203 {
          selector: w203 -> [_ w210 _ w232 w241 _]
          tunnel: w200 -> [_ _ w229 w231 _ w248]
          tunnel: cluster{string[]}[] [{["640x480", "320x240", "160x120"]}, {["Auto", "Fixed indoor", "Fixed outdoor 1", "Fixed outdoor 2", "Fixed fluorescent 1", "Fixed fluorescent 2", "Hold current"]}, {["Auto", "Flicker-free 50 Hz", "Flicker-free 60 Hz", "Hold current"]}, {["None", "Prioritize frame rate", "Prioritize image quality"]}, {["Monochrome", "Color"]}] -> [_ _ _ _ _ w247]
          frame Default {
            w205 = FALSE ("Visible")
            w204 = FALSE ("Visible")
            n115 = property on="Motor" class="Clust (strict)"("Visible"=w204) -> ()  [unwired: 2 in, 2 out]
            n116 = property on="Test Ring" class="Ring (strict)"("Visible"=w204) -> ()  [unwired: 2 in, 2 out]
            n117 = property on="Rev/Fwd" class="Clust (strict)"("Visible"=w205) -> ()  [unwired: 2 in, 2 out]
            n118 = property on="On/Off" class="Bool (strict)"("Visible"=w205) -> ()  [unwired: 2 in, 2 out]
            n119 = property on="Test Slider" class="Slide (strict)"("Visible"=w205) -> ()  [unwired: 2 in, 2 out]
          }
          frame "Analog Out", "Motor", "PWM" {
            w211 = FALSE ("Visible")
            n120 = case shown="\"Analog Out\"" w210 {
              tunnel: [1.0 ("Value") -1.0 ("Value") 0.0 ("Value")] -> w209
              tunnel: [255.0 ("Value") 1.0 ("Value") 5.0 ("Value")] -> w208
              tunnel: [128.0 ("Value") 0.0 ("Value") 0.0 ("Value")] -> w207
              tunnel: [64.0 ("Value") 0.5 ("Value") 1.0 ("Value")] -> w206
              frame "PWM" {
              }
              frame "Motor", Default {
              }
              frame "Analog Out" {
              }
            }
            n121 = property on="Motor" class="Clust (strict)"("Visible"=TRUE) -> ()  [unwired: 2 in, 2 out]
            n122 = property on="Value" class="Slide (strict)"("Value"=w207, "Scale.Minimum"=w209, "Scale.Maximum"=w208, "Scale.Increment"=w206) -> ()  [unwired: 2 in, 2 out]
            n123 = property on="On/Off" class="Bool (strict)"("Visible"=w211) -> ()  [unwired: 2 in, 2 out]
            n124 = property on="Test Slider" class="Slide (strict)"("Visible"=w211) -> ()  [unwired: 2 in, 2 out]
            n125 = property on="Test Ring" class="Ring (strict)"("Visible"=w211) -> ()  [unwired: 2 in, 2 out]
            n126 = property on="Rev/Fwd" class="Clust (strict)"("Visible"=w211) -> ()  [unwired: 2 in, 2 out]
          }
          frame "Servo" {
            w227 = FALSE ("Visible")
            n127 = call <vilib>:"NT Read Number.vi"("Name"=w229) -> ("Numeric"=w228:dbl)  [unwired: 9 in, 1 out]
            n128 = property on="Test Slider" class="Slide (strict)"("Visible"=TRUE, "Scale.Maximum"=170.0 ("Scale.Range:Maximum")) -> ()  [unwired: 2 in, 2 out]
            n129 = local write "Test Slider"(w228) -> ()
            n130 = property on="Motor" class="Clust (strict)"("Visible"=w227) -> ()  [unwired: 2 in, 2 out]
            n131 = property on="Rev/Fwd" class="Clust (strict)"("Visible"=w227) -> ()  [unwired: 2 in, 2 out]
            n132 = property on="On/Off" class="Bool (strict)"("Visible"=w227) -> ()  [unwired: 2 in, 2 out]
            n133 = property on="Test Ring" class="Ring (strict)"("Visible"=w227) -> ()  [unwired: 2 in, 2 out]
          }
          frame "Relay", "Solenoid" {
            w230 = FALSE ("Visible")
            n134 = property on="Motor" class="Clust (strict)"("Visible"=w230) -> ()  [unwired: 2 in, 2 out]
            n135 = property on="Test Slider" class="Slide (strict)"("Visible"=w230) -> ()  [unwired: 2 in, 2 out]
            n136 = Search and Replace String(input string=w231, search string="/Value  **", replace string="/Direction") -> (result string=w237:string)  [unwired: 5 in, 3 out]
            n137 = property on="Test Ring" class="Ring (strict)"("Visible"=w230) -> ()  [unwired: 2 in, 2 out]
            n138 = call <vilib>:"NT Read String.vi"("Name"=w237) -> ("String"=w235:string)  [unwired: 9 in, 1 out]
            n139 = Equal?(x="Both directions", y=w235) -> (x = y?=w233:bool)
            n140 = Not(x=w233) -> (.not. x?=w234:bool)
            n141 = property on="Rev/Fwd" class="Clust (strict)"("Visible"=w233) -> ()  [unwired: 2 in, 2 out]
            n142 = property on="On/Off" class="Bool (strict)"("Visible"=w234, "Caption.Text"=w232) -> ()  [unwired: 2 in, 2 out]
          }
          frame "Compressor", "Digital Out" {
            w240 = FALSE ("Visible")
            # "Get direction and finish"
            n143 = property on="Motor" class="Clust (strict)"("Visible"=w240) -> ()  [unwired: 2 in, 2 out]
            n144 = property on="Test Slider" class="Slide (strict)"("Visible"=w240) -> ()  [unwired: 2 in, 2 out]
            n145 = property on="Test Ring" class="Ring (strict)"("Visible"=w240) -> ()  [unwired: 2 in, 2 out]
            n146 = property on="On/Off" class="Bool (strict)"("Visible"=TRUE, "Caption.Text"=w241) -> ()  [unwired: 2 in, 2 out]
            n147 = property on="Rev/Fwd" class="Clust (strict)"("Visible"=FALSE) -> ()  [unwired: 2 in, 2 out]
          }
          frame "Camera" {
            n148 = call <vilib>:"Get Last Path Segment.vi"("String in"=w248) -> ("String out"=w249:string)  [unwired: 10 in]
            n149 = property on="On/Off" class="Bool (strict)"("Visible"=FALSE) -> ()  [unwired: 2 in, 2 out]
            n150 = property on="Motor" class="Clust (strict)"("Visible"=FALSE) -> ()  [unwired: 2 in, 2 out]
            n151 = property on="Rev/Fwd" class="Clust (strict)"("Visible"=FALSE) -> ()  [unwired: 2 in, 2 out]
            n152 = case shown="\"White Balance  **\"" w249 {
              tunnel: w248 -> [w255 w264 w273 w282 w291 _ w297]
              tunnel: w247 -> [w253 w261 w270 w279 w288 _ _]
              frame "Size  **" {
                n153 = Index Array(array=w253) -> (element=w252:cluster{string[]})  [unwired: 1 in]
                n154 = call <vilib>:"NT Read String.vi"("Name"=w255) -> ("String"=w254:string)  [unwired: 9 in, 1 out]
                n155 = Unbundle(w252) -> (w250:string[])
                n156 = Match First String(2:w250, 3:w254) -> (0:w251:i32)  [unwired: 1 out]
                n157 = property on="Test Ring" class="Ring (strict)"("Value"=w251, "Strings []"=w250) -> ()  [unwired: 2 in, 2 out]
                n158 = property on="Test Ring" class="Ring (strict)"("Visible"=TRUE) -> ()  [unwired: 2 in, 2 out]
                n159 = property on="Test Slider" class="Slide (strict)"("Visible"=FALSE) -> ()  [unwired: 2 in, 2 out]
              }
              frame "White Balance  **" {
                n160 = Index Array(array=w261, index=1) -> (element=w262:cluster{string[]})
                n161 = call <vilib>:"NT Read String.vi"("Name"=w264) -> ("String"=w263:string)  [unwired: 9 in, 1 out]
                n162 = Unbundle(w262) -> (w259:string[])
                n163 = Match First String(2:w259, 3:w263) -> (0:w258:i32)  [unwired: 1 out]
                n164 = property on="Test Ring" class="Ring (strict)"("Value"=w258, "Strings []"=w259) -> ()  [unwired: 2 in, 2 out]
                n165 = property on="Test Ring" class="Ring (strict)"("Visible"=TRUE) -> ()  [unwired: 2 in, 2 out]
                n166 = property on="Test Slider" class="Slide (strict)"("Visible"=FALSE) -> ()  [unwired: 2 in, 2 out]
              }
              frame "Exposure  **" {
                n167 = Index Array(array=w270, index=2) -> (element=w271:cluster{string[]})
                n168 = call <vilib>:"NT Read String.vi"("Name"=w273) -> ("String"=w272:string)  [unwired: 9 in, 1 out]
                n169 = Unbundle(w271) -> (w267:string[])
                n170 = Match First String(2:w267, 3:w272) -> (0:w268:i32)  [unwired: 1 out]
                n171 = property on="Test Ring" class="Ring (strict)"("Value"=w268, "Strings []"=w267) -> ()  [unwired: 2 in, 2 out]
                n172 = property on="Test Ring" class="Ring (strict)"("Visible"=TRUE) -> ()  [unwired: 2 in, 2 out]
                n173 = property on="Test Slider" class="Slide (strict)"("Visible"=FALSE) -> ()  [unwired: 2 in, 2 out]
              }
              frame "Exposure Priority  **" {
                n174 = Index Array(array=w279, index=3) -> (element=w280:cluster{string[]})
                n175 = call <vilib>:"NT Read String.vi"("Name"=w282) -> ("String"=w281:string)  [unwired: 9 in, 1 out]
                n176 = Unbundle(w280) -> (w276:string[])
                n177 = Match First String(2:w276, 3:w281) -> (0:w277:i32)  [unwired: 1 out]
                n178 = property on="Test Ring" class="Ring (strict)"("Value"=w277, "Strings []"=w276) -> ()  [unwired: 2 in, 2 out]
                n179 = property on="Test Ring" class="Ring (strict)"("Visible"=TRUE) -> ()  [unwired: 2 in, 2 out]
                n180 = property on="Test Slider" class="Slide (strict)"("Visible"=FALSE) -> ()  [unwired: 2 in, 2 out]
              }
              frame "Color Enable  **" {
                n181 = Index Array(array=w288, index=4) -> (element=w289:cluster{string[]})
                n182 = call <vilib>:"NT Read String.vi"("Name"=w291) -> ("String"=w290:string)  [unwired: 9 in, 1 out]
                n183 = Unbundle(w289) -> (w285:string[])
                n184 = Match First String(2:w285, 3:w290) -> (0:w286:i32)  [unwired: 1 out]
                n185 = property on="Test Ring" class="Ring (strict)"("Value"=w286, "Strings []"=w285) -> ()  [unwired: 2 in, 2 out]
                n186 = property on="Test Ring" class="Ring (strict)"("Visible"=TRUE) -> ()  [unwired: 2 in, 2 out]
                n187 = property on="Test Slider" class="Slide (strict)"("Visible"=FALSE) -> ()  [unwired: 2 in, 2 out]
              }
              frame Default {
                n188 = property on="Test Ring" class="Ring (strict)"("Visible"=FALSE) -> ()  [unwired: 2 in, 2 out]
                n189 = property on="Test Slider" class="Slide (strict)"("Visible"=FALSE) -> ()  [unwired: 2 in, 2 out]
              }
              frame "Brightness  **", "Color Level  **", "Compression  **", "FPS  **", "Sharpness  **" {
                n190 = call <vilib>:"NT Read Number.vi"("Name"=w297) -> ("Numeric"=w296:dbl)  [unwired: 9 in, 1 out]
                n191 = local write "Test Slider"(w296) -> ()
                n192 = property on="Test Slider" class="Slide (strict)"("Visible"=TRUE, "Scale.Maximum"=100.0 ("Scale.Range:Maximum")) -> ()  [unwired: 2 in, 2 out]
                n193 = property on="Test Ring" class="Ring (strict)"("Visible"=FALSE) -> ()  [unwired: 2 in, 2 out]
              }
            }
          }
        }
        n194 = property on="Progress" class="Clust (strict)"("Visible"=FALSE) -> ()  [unwired: 2 in, 2 out]
      }
      event "Test Name": Mouse Enter {
        # "Populate the ring with the list of tests"
        n195 = event-data() -> ()  [unwired: 1 in, 1 out]
        n196 = call <vilib>:"NT Read String Array.vi"("Name"="TestMode/TestList") -> ("String Array"=w305:string[])  [unwired: 9 in, 1 out]
        n197 = Build Array (concatenate)("Select the test to run...", w305) -> (w304:string[])
        n198 = property on="Test Name" class="Ring (strict)"("Strings []"=w304) -> ()  [unwired: 2 in, 2 out]
      }
      event "Test Name": Value Change {
        w307 = FALSE ("Visible")
        # "Tell the robot the test name to run"
        n199 = event-data() -> ("NewVal"=w311:u16)  [unwired: 1 in]
        n200 = property on="Test Name" class="Ring (strict)"() -> ("Strings []"=w312:string[])  [unwired: 2 in, 2 out]
        n201 = local write "Progress"(T6 {"Test Progress"=0, "Test Progress Text"=""} ("Progress")) -> ()
        n202 = Index Array(array=w312, index=w311) -> (element=w310:string)
        n203 = call <vilib>:"NT Write String.vi"("String"=w310, "Name"="TestMode/TestName") -> ()  [unwired: 9 in, 1 out]
        n204 = property on="Progress" class="Clust (strict)"("Visible"=TRUE) -> ()  [unwired: 2 in, 2 out]
        n205 = property on="Motor" class="Clust (strict)"("Visible"=w307) -> ()  [unwired: 2 in, 2 out]
        n206 = property on="Test Slider" class="Slide (strict)"("Visible"=w307) -> ()  [unwired: 2 in, 2 out]
        n207 = property on="On/Off" class="Bool (strict)"("Visible"=w307) -> ()  [unwired: 2 in, 2 out]
        n208 = property on="Rev/Fwd" class="Clust (strict)"("Visible"=w307) -> ()  [unwired: 2 in, 2 out]
        n209 = property on="Test Ring" class="Ring (strict)"("Visible"=w307) -> ()  [unwired: 2 in, 2 out]
      }
      event "Select Auto": Mouse Enter {
        # "Populate the combo box with the list of autonomous options"
        n210 = event-data() -> ()  [unwired: 1 in, 1 out]
        n211 = call <vilib>:"NT Read String Array.vi"("Name"="Auto List") -> ("String Array"=w314:string[])  [unwired: 9 in, 1 out]
        n212 = property on="Select Auto" class="CmbBox"("Strings[]"=w314) -> ()  [unwired: 2 in, 2 out]
      }
      event "Select Auto": Value Change {
        # "User modified the Auto Selection. Write to NT variable so robot knows."
        n213 = event-data() -> ("NewVal"=w317:string)  [unwired: 1 in]
        n214 = call <vilib>:"NT Write String.vi"("String"=w317, "Name"="Auto Selector") -> ()  [unwired: 9 in, 1 out]
      }
      event "Command Selection": Value Change {
        # "Get the params and show in table"
        n215 = event-data() -> ("NewVal"=w323:i32)  [unwired: 1 in]
        n216 = property on="Command Selection" class="MCListbox (strict)"() -> ("ItemNames"=w321:string[][])  [unwired: 2 in, 2 out]
        n217 = call <vilib>:"WPI_DashboardUpdate Command Params.vi"("NewVal"=w323, "Commands"=w321, "Param Tbl"=w322) -> ()  [unwired: 8 in, 1 out]
      }
      event "Execute Command": Value Change {
        # "Started one, Unique ID holds\nresponse"
        n218 = event-data() -> ()  [unwired: 1 in, 1 out]
        n219 = property on="Command Selection" class="MCListbox (strict)"() -> ("ItemNames"=w334:string[][])  [unwired: 2 in, 2 out]
        n220 = Index Array(array=w334, index (row)="Command Selection", index (col)=0) -> (element=w332:string)
        n221 = call <vilib>:"Invoke Commands.vi"("Command Params"="Command Params", "Function Name"=w332) -> ("Params"=w328:u8, "Started"=w327:bool)  [unwired: 7 in, 1 out]
        n222 = Array Subset(array="Command Params", length (row)=w328) -> (w329:string[][])  [unwired: 3 in]
        n223 = Select(t="Executing" ("Cmd Status"), s=w327, f="" ("Cmd Status")) -> (s? t:f=→"Cmd Status":string)
      }
      event "Command Selection": Double Click {
        n224 = event-data() -> ("Row"=w342:i32)  [unwired: 1 in]
        n225 = property on="Command Selection" class="MCListbox (strict)"() -> ("ItemNames"=w345:string[][])  [unwired: 2 in, 2 out]
        n226 = local read "Command Params"() -> (w341:string[][])
        n227 = Index Array(array=w345, index (row)=w342, index (col)=0) -> (element=w343:string)
        n228 = call <vilib>:"Invoke Commands.vi"("Command Params"=w341, "Function Name"=w343) -> ("Params"=w340:u8, "Started"=w335:bool)  [unwired: 7 in, 1 out]
        n229 = Array Subset(array=w341, length (row)=w340) -> (w339:string[][])  [unwired: 3 in]
        n230 = Select(t="Executing" ("Cmd Status"), s=w335, f="" ("Cmd Status")) -> (s? t:f=w336:string)
        n231 = local write "Cmd Status"(w336) -> ()
      }
      event "CheckList": Double Click {
        # "Shift clears all"
        # "Update symbols on the listbox"
        n232 = event-data() -> ("PlatMods.Shift"=w347:bool, "Row"=w349:i32)  [unwired: 1 in]
        n233 = case shown="True" w347 {
          tunnel: w349 -> [w353 _]
          tunnel: 1 -> [w352 _]
          frame False {
            n234 = property on="CheckList" class="LstBox (strict)"() -> ("Item Symbols"=w351:i32[])  [unwired: 2 in, 2 out]
            n235 = Replace Array Subset(array=w351, new element=w352, index=w353) -> (w350:i32[])
            n236 = property on="CheckList" class="LstBox (strict)"("Item Symbols"=w350) -> ()  [unwired: 2 in, 2 out]
          }
          frame True {
            w354 = 0 ("Top Row")
            n237 = property on="CheckList" class="LstBox (strict)"() -> ("Number of Rows"=w356:u32)  [unwired: 2 in, 2 out]
            n238 = Initialize Array(0, w356) -> (w355:i32[])
            n239 = property on="CheckList" class="LstBox (strict)"("Top Row"=w354, "Value"=w354, "Item Symbols"=w355) -> ()  [unwired: 2 in, 2 out]
          }
        }
      }
      event "CheckList": Key Down {
        # "Update symbols on the listbox\nLeft and right keys check and uncheck"
        n240 = event-data() -> ("VKey"=w360:T15)  [unwired: 1 in]
        n241 = case shown="\"Left\", \"Right\"" w360 {
          selector: w360 -> [w365 _]
          tunnel: eventvkey."Left" ("VKey") -> [w363 _]
          frame "Left", "Right" {
            n242 = Equal?(x=w363, y=w365) -> (x = y?=w364:bool)
            n243 = Select(t=0, s=w364, f=1) -> (s? t:f=w366:i32)
            n244 = property on="CheckList" class="LstBox (strict)"() -> ("Item Symbols"=w369:i32[])  [unwired: 2 in, 2 out]
            n245 = Replace Array Subset(array=w369, new element=w366, index="CheckList") -> (w368:i32[])
            n246 = property on="CheckList" class="LstBox (strict)"("Item Symbols"=w368) -> ()  [unwired: 2 in, 2 out]
          }
          frame Default {
          }
        }
      }
      event "Motor.Enable": Value Change {
        # "When the test mode otor enable helper is set, update that\ntree row item's value"
        n247 = event-data() -> ("NewVal"=w375:bool)  [unwired: 1 in]
        n248 = Unbundle("Motor") -> ("Value"=w374:dbl)  [unwired: 1 out]
        n249 = Select(t=w374, s=w375, f=0.0) -> (s? t:f=w372:dbl)
        n250 = call <vilib>:"NT Write Number.vi"("Numeric"=w372, "Name"=w371) -> ()  [unwired: 9 in, 1 out]
      }
      event "Test Slider": Value Change {
        # "When the test mode slider helper is set, update that\ntree row item's value"
        n251 = event-data() -> ("NewVal"=w378:dbl)  [unwired: 1 in]
        n252 = call <vilib>:"NT Write Number.vi"("Numeric"=w378, "Name"=w379) -> ()  [unwired: 9 in, 1 out]
      }
      event "On/Off": Value Change {
        # "When the test mode on/off helper value is set, update that\ntree row item's value"
        n253 = event-data() -> ("NewVal"=w383:bool)  [unwired: 1 in]
        n254 = Boolean To (0,1)(Boolean=w383) -> (0, 1=w382:i16)
        n255 = call <vilib>:"NT Write Number.vi"("Numeric"=w382, "Name"=w381) -> ()  [unwired: 9 in, 1 out]
      }
      event "Rev/Fwd": Value Change {
        # "When the test mode helper value for relays is set, update that\ntree row item's value"
        n256 = event-data() -> ("NewVal.Forward"=w391:bool, "NewVal.Reverse"=w390:bool)  [unwired: 1 in]
        n257 = Boolean To (0,1)(Boolean=w391) -> (0, 1=w387:i16)
        n258 = Boolean To (0,1)(Boolean=w390) -> (0, 1=w389:i16)
        n259 = Negate(x=w389) -> (-x=w388:i16)
        n260 = Add(x=w387, y=w388) -> (x+y=w386:i16)
        n261 = call <vilib>:"NT Write Number.vi"("Numeric"=w386, "Name"=w385) -> ()  [unwired: 9 in, 1 out]
      }
      event "Test Ring": Value Change {
        # "When a test mode helper value is selected from the ring,\nset the tree item's variable to the string value"
        n262 = event-data() -> ("NewVal"=w395:u16)  [unwired: 1 in]
        n263 = property on="Test Ring" class="Ring (strict)"() -> ("Strings []"=w396:string[])  [unwired: 2 in, 2 out]
        n264 = Index Array(array=w396, index=w395) -> (element=w394:string)
        n265 = call <vilib>:"NT Write String.vi"("String"=w394, "Name"=w393) -> ()  [unwired: 9 in, 1 out]
      }
      event "Rec Mode": Value Change {
        # "Update globals for recording mode and path to read log from.\nClear when logging and let NetworkTables set path for vision to\nuse."
        n266 = event-data() -> ("NewVal"=w407:enum32{"Stop", "Record", "Playback"})  [unwired: 1 in]
        n267 = global write "WPI_DashboardLogging Global.vi" "Logging Filename"(path "") -> ()
        n268 = global write "WPI_DashboardLogging Global.vi" "Recording"(w407) -> ()
        n269 = case shown="\"Playback\"" w407 {
          tunnel: w406 -> [_ w409 w418]
          tunnel: [_ _ w417] -> w404
          tunnel: [_ _ w416] -> _
          tunnel: w402 -> [_ _ w414]
          tunnel: cluster{i32, i32} {-250, 170} -> [_ _ w413]
          tunnel: [_ _ T16 {"Image Size"=TRUE, "Image Type"=TRUE, "Pixel Value"=TRUE, "ROI Information"=TRUE, "Zoom Factor"=FALSE} ("Image Information Shown:All Elements")] -> w397
          tunnel: [_ _ TRUE ("Zoom Factor")] -> w398
          tunnel: w400 -> [_ _ w410]
          frame Default {
          }
          frame "Stop", "Record" {
            # "Place Window too"
            n270 = invoke class="VI" method="FP.Close"(reference=w409) -> (reference out=w408:refnum<vi>)  [unwired: 2 in, 2 out]
            n271 = invoke class="VI" method="Abort VI"(reference=w408) -> ()  [unwired: 2 in, 3 out]
          }
          frame "Playback" {
            n272 = call "Open Playback Panel.vi"("Offset"=w413, "DB VI Ref"=w414, "Playback in"=w418) -> ("Playback out"=w415:refnum<vi>)  [unwired: 8 in]
            n273 = register-events(w415, w410) -> (reference out=w417:refnum<event-registration>, error out=w416:errorcluster)  [unwired: 2 in]
          }
        }
        n274 = property on="Camera Image Right" class="ImageControl"("Image Information Shown"=w397, "Image Information Visible"=w398) -> ()  [unwired: 2 in, 2 out]
        n275 = property on="Camera Image" class="ImageControl"("Image Information Shown"=w397, "Image Information Visible"=w398) -> ()  [unwired: 2 in, 2 out]
        n276 = call <vilib>:"WPI_DashboardNT Log FieldName Cache.vi"("Operation"=enum16{"Lookup/Add", "Index", "Clear"}."Clear") -> ()  [unwired: 8 in, 3 out]
      }
      event Panel Close {
        w420 = enum32{"Stop", "Record", "Playback"}."Stop" ("Rec Mode")
        # "Playback window has been closed, abort"
        n277 = event-data() -> ()  [unwired: 1 in, 4 out]
        n278 = local write "Rec Mode"(w420) -> ()
        n279 = global write "WPI_DashboardLogging Global.vi" "Recording"(w420) -> ()
      }
      event Panel Close {
        # "Abort playback window and ourself"
        n280 = event-data() -> ()  [unwired: 1 in, 4 out]
        n281 = invoke class="VI" method="FP.Close"(reference=w424) -> (reference out=w423:refnum<vi>)  [unwired: 2 in, 2 out]
        n282 = invoke class="VI" method="Abort VI"(reference=w423) -> (error out=w422:errorcluster)  [unwired: 2 in, 2 out]
        n283 = invoke class="VI" method="Abort VI"(error in=w422) -> ()  [unwired: 2 in, 3 out]
      }
      event User Event {
        n284 = event-data() -> ("IDs"=w431:cluster{"RPC field ID":u16, "Unique ID":u16}, "String"=w430:string)  [unwired: 1 in]
        n285 = Bundle("IDs"=w431, "String"=w430) -> (w429:T9)  [unwired: 1 in]
        n286 = call <vilib>:"Retrieve RPC Response.vi"("RPC Response"=w429) -> ("Output"=w427:string[][])  [unwired: 10 in]
        n287 = Build Array (concatenate)(w425, w427) -> (w426:string[][])
        n288 = local write "Command Params"(w426) -> ()
        n289 = local write "Cmd Status"("" ("Cmd Status")) -> ()
      }
      event "Tree": Double Click {
        n290 = event-data() -> ("PlatMods"=w437:T19, "Tag"=w434:string)  [unwired: 1 in]
        n291 = Unbundle(w437) -> ("Shift"=w436:bool)  [unwired: 4 out]
        n292 = String Subset(string=w434, length (rest)=1 ("length (rest)")) -> (substring=w433:string)  [unwired: 1 in]
        n293 = Not(x=w436) -> (.not. x?=w435:bool)
        n294 = case shown="\"/\"" w433 {
          tunnel: w434 -> [_ w440]
          tunnel: w435 -> [_ w439]
          frame Default {
          }
          frame "/" {
            n295 = call <vilib>:"NT Update Persistence.vi"("Persistence"=w439, "Name"=w440) -> ()  [unwired: 9 in, 1 out]
          }
        }
      }
    }
  }
  n296 = while {
    tunnel: w66 -> [w442]
    i -> [w445]
    stop <- FALSE stop-if-true
    n297 = Wait (ms)(milliseconds to wait=u32 100) -> ()  [unwired: 1 out]
    n298 = case shown="\"Playback\"" "Rec Mode" {
      tunnel: w445 -> [_ _ w460]
      tunnel: [u32 2829099 ("Base Color") u32 11141120 ("Target Color") w449] -> w441
      frame "Stop", Default {
        # "Reset the color, extra updates don't cost much"
      }
      frame "Record" {
      }
      frame "Playback" {
        # "Playback"
        n299 = Quotient & Remainder(x=w460, y=u32 50 ("milliseconds to wait")) -> (x-y*floor(x/y)=w456:u32)  [unwired: 1 out]
        n300 = Divide(x=w456, y=u32 50 ("milliseconds to wait")) -> (x/y=w453:dbl)
        n301 = Multiply(x=6.283185307179586, y=w453) -> (x*y=w458:dbl)
        n302 = Sine(x=w458) -> (sin(x)=w457:dbl)
        n303 = Absolute Value(x=w457) -> (abs(x)=w450:dbl)
        n304 = call "Interpolate RGB Color.vi"("Proportion"=w450, "Target Color"=u32 30976, "Base Color"=u32 2829099) -> ("Result Color"=w449:u32)  [unwired: 8 in]
      }
    }
    n305 = property class="Pane"(reference=w442, "PaneColor"=w441) -> ()  [unwired: 1 in, 2 out]
  }
  n306 = local write "Dashboard Tab"(T2."Drive" ("Dashboard Tab")) -> ()
  n307 = property on="On/Off" class="Bool (strict)"("Visible"=w37) -> ()  [unwired: 2 in, 2 out]
  n308 = property on="Motor" class="Clust (strict)"("Visible"=w37) -> ()  [unwired: 2 in, 2 out]
  n309 = property on="Progress" class="Clust (strict)"("Visible"=w37) -> ()  [unwired: 2 in, 2 out]
  n310 = property on="Test Ring" class="Ring (strict)"("Visible"=w37) -> ()  [unwired: 2 in, 2 out]
  n311 = property on="Rev/Fwd" class="Clust (strict)"("Visible"=w37) -> ()  [unwired: 2 in, 2 out]
  n312 = while {
    tunnel: u16 1741 ("timeout ms (25000)") -> [w462]
    stop <- FALSE stop-if-true
    n313 = TCP Create Listener(10:w462) -> (0:w461:errorcluster, 3:w463:refnum<k5>)  [unwired: 4 in, 1 out]
    n314 = case shown="No Error" w461 {
      selector: w461 -> [w465 _]
      tunnel: w463 -> [w466 _]
      frame No Error {
        n315 = while {
          tunnel: w466 -> [w469]
          tunnel: w465 -> [w468]
          stop <- FALSE stop-if-true
          n316 = TCP Wait On Listener(8:w468, 11:w469) -> (0:w470:errorcluster, 4:w471:refnum<k5>)  [unwired: 2 in, 3 out]
          n317 = local write "TCP"(w471) -> ()
          n318 = case shown="No Error" w470 {
            frame No Error {
            }
            frame Error {
              n319 = Wait (ms)(milliseconds to wait=u32 1000) -> ()  [unwired: 1 out]
            }
          }
        }
      }
      frame Error {
        n320 = Wait (ms)(milliseconds to wait=u32 1000) -> ()  [unwired: 1 out]
      }
    }
  }
  n321 = call <vilib>:"Intialize Keyboard.vi"() -> ("device ID"=w1:refnum<k1>)  [unwired: 10 in, 1 out]
  n322 = while {
    tunnel: [w484] -> _
    tunnel: w36 -> [w478]
    tunnel: w35 -> [w475]
    tunnel: w1 -> [w474]
    i -> [w484]
    stop <- FALSE stop-if-true
    n323 = call <vilib>:"WPI_DashboardRetrieveStatusInfo.vi"("Binding Refnum"=w478, "Window Mode Notifier"=w475, "TCP Cnx"="TCP") -> ("Power and Errors"=w479:T20, "Robot Metrics"=w482:T21, "Status Info"=w483:T22, "Control Info"=w480:T23, "Robot Mode"=w477:T4, "Process?"=w481:bool)  [unwired: 3 in]
    "Mode" <- w477
    n324 = case shown="True" w481 {
      tunnel: w483 -> [_ w522]
      tunnel: w482 -> [_ w521]
      tunnel: w480 -> [_ w520]
      tunnel: w479 -> [_ w519]
      tunnel: w477 -> [_ _]
      tunnel: w474 -> [_ w490]
      frame False {
        n325 = Wait (ms)(milliseconds to wait=u32 20) -> ()  [unwired: 1 out]
      }
      frame True {
        # "swap motors to match\ncharts and include battery"
        n326 = Unbundle By Name(w520) -> ("Joystick Values"=w505:T24)  [unwired: 1 out]
        n327 = Unbundle By Name(w521) -> ()  [unwired: 1 out]
        n328 = Unbundle By Name(w519) -> ("Robot IP"=→"Robot IP":string)
        n329 = Unbundle By Name(w522) -> ()  [unwired: 2 out]
        n330 = control-ref of="XY Graph"() -> (w495:refnum<vi>)
        n331 = call-poly <vilib>:"NT Read Value.vi"("Name"="RobotDrive Motors") -> ("Numeric Array"=w507:dbl[])  [unwired: 9 in, 1 out]
        n332 = Index Array(array=w507, index #1=1, index #4=0) -> (element #1=w514:dbl, element #2=w515:dbl, element #3=w513:dbl, element #4=w518:dbl)  [unwired: 2 in]
        n333 = Index Array(array=w505) -> (element=w492:T25)  [unwired: 1 in]
        n334 = Unbundle By Name(w492) -> ("Axes"=w493:dbl[])  [unwired: 1 out]
        n335 = call "Dashboard Cursor Interpolation.vi"("Remove Cursor"="Remove Point", "Add Cursor"="Add Point", "Joystick Input"=w493, "Graph Detail"=500, "Interpolation Method"="Interpolation Method", "Interpolation Points"=w495) -> ("Joystick Output"=w499:dbl[])  [unwired: 5 in]
        n336 = Index Array(array=w499) -> (element #1=w500:dbl, element #2=w501:dbl, element #3=→"JS2 Z":dbl)  [unwired: 3 in]
        n337 = Bundle("Numeric"=w500, "Numeric"=w501) -> (w502:cluster{"Numeric":dbl, "Numeric":dbl})  [unwired: 1 in]
        n338 = Build Array(w502) -> (→"JS2 Graph":cluster{"Numeric":dbl, "Numeric":dbl}[])
        n339 = Bundle("Numeric"=w513, "Numeric"=w514) -> (→"MotorChart R" →"MotorSliders R":cluster{"Numeric":dbl, "Numeric":dbl})  [unwired: 1 in]
        n340 = Bundle("Numeric"=w515, "Numeric"=w518) -> (→"MotorChart L" →"MotorSliders L":cluster{"Numeric":dbl, "Numeric":dbl})  [unwired: 1 in]
        n341 = call "Prepare Joystick Data for Displays.vi"("Joystick Values"=w492) -> ("Buttons"=→"JS1 Buttons" →"JS2 Buttons":T26, "Z Axis"=→"JS1 Z":dbl, "Cartesian Data"=→"JS1 Graph":cluster{"X axis":dbl, "X axis":dbl}[])  [unwired: 8 in]
        n342 = call-poly <vilib>:"Acquire Input Data.vi"("device ID"=w490) -> ("keys pressed"=w489:T27)  [unwired: 16 in, 2 out]
        n343 = Index Array(array=w489) -> (element=w488:T28)  [unwired: 1 in]
        n344 = call-poly <vilib>:"NT Write Value.vi"("Numeric"=w488, "Name"="Keyboard Data") -> ()  [unwired: 9 in, 1 out]
      }
    }
  }
  n345 = local write "Command Selection"(u16 0 ("milliseconds to wait")) -> ()
  n346 = local write "Command Params"(string[][] [] ("Command Params")) -> ()
  n347 = global write "WPI_DashboardLogging Global.vi" "Recording"(w60) -> ()
  n348 = local write "Rec Mode"(w60) -> ()
  n349 = call <vilib>:"NT Write String.vi"("String"="Select Auto", "Name"="Auto Selector") -> ()  [unwired: 9 in, 1 out]
